vi "Scroll_Pump_Monitoring_Manipulate_Parameters.vi"(0 "FGGA_Scroll_Pump\nMonitoring_Input":string[](array[string])) -> (4 "output array":string[](array[string]))   [LabVIEW 2014]
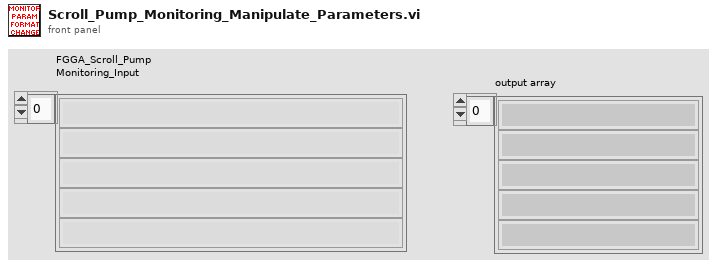
[diagram p1: front panel]
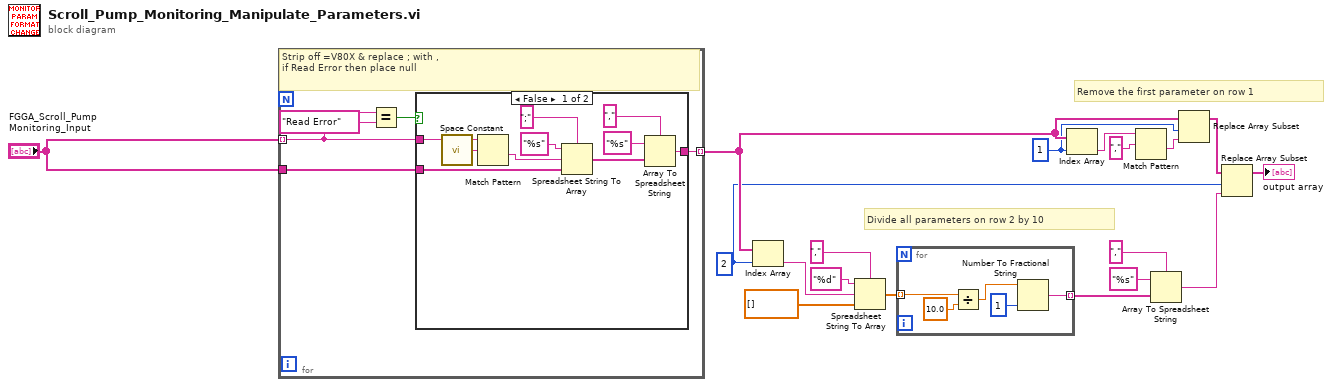
[diagram p0: block diagram]
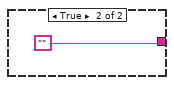
[diagram p2: hidden frame]
diagram:
  w3 = 2 ("index")
  w6 = 1 ("index")
  # "Divide all parameters on row 2 by 10"
  # "Remove the first parameter on row 1"
  n1 = for {
    tunnel: "FGGA_Scroll_Pump\nMonitoring_Input" -> [w23]
    tunnel: "FGGA_Scroll_Pump\nMonitoring_Input" -> [w21] mode=indexing
    tunnel: [w22] -> w7 mode=indexing
    # "Strip off =V80X & replace ; with ,\nif Read Error then place null"
    n2 = Equal?(x=w21, y="Read Error") -> (x = y?=w19:bool)
    n3 = case shown="False" w19 {
      tunnel: w23 -> [w29 _]
      tunnel: w21 -> [w25 _]
      tunnel: [w24 ""] -> w22
      frame False {
        n4 = call <vilib>:"Space Constant.vi"() -> ("String"=w33:string)
        n5 = Match Pattern(string=w25, regular expression=w33) -> (after substring=w32:string)  [unwired: 1 in, 3 out]
        n6 = Spreadsheet String To Array(delimiter (Tab)=";", format string="%s", spreadsheet string=w32, array type (2D Dbl)=w29) -> (array=w28:string[])
        n7 = Array To Spreadsheet String(delimiter (Tab)=",", array=w28, 3:"%s" ("format string")) -> (spreadsheet string=w24:string)
      }
      frame True {
      }
    }
  }
  n8 = Index Array(array=w7, index=w3) -> (element=w13:string)
  n9 = Spreadsheet String To Array(delimiter (Tab)=",", format string="%d", spreadsheet string=w13, array type (2D Dbl)=dbl[] []) -> (array=w11:dbl[])
  n10 = for {
    tunnel: w11 -> [w39] mode=indexing
    tunnel: [w35] -> w8 mode=indexing
    n11 = Divide(x=w39, y=10.0) -> (x/y=w37:dbl)
    n12 = Number To Fractional String(number=w37, precision (6)=i16 1) -> (F-format string=w35:string)  [unwired: 2 in]
  }
  n13 = Index Array(array=w7, index=w6) -> (element=w18:string)
  n14 = Match Pattern(string=w18, regular expression=",") -> (after substring=w5:string)  [unwired: 1 in, 3 out]
  n15 = Array To Spreadsheet String(delimiter (Tab)=",", array=w8, 3:"%s" ("format string")) -> (spreadsheet string=w2:string)
  n16 = Replace Array Subset(array=w7, new element=w5, index=w6) -> (w4:string[])
  n17 = Replace Array Subset(array=w4, new element=w2, index=w3) -> (→"output array":string[])
